vi "BinCoincidence.vi"(2 "lateral peaks":u32, 3 "rawdata":T1, 4 "center peak (µs)":dbl format="%.2f", 5 "delay channel":i32, 6 "histogram lenght (µs)":dbl format="%.2f", 7 "binning":dbl format="%.2f") -> (0 "center peak trace":u32[](array[numeric]), 1 "coincidence trace":dbl[](array[numeric]) format="%.2f")   [LabVIEW 2009]
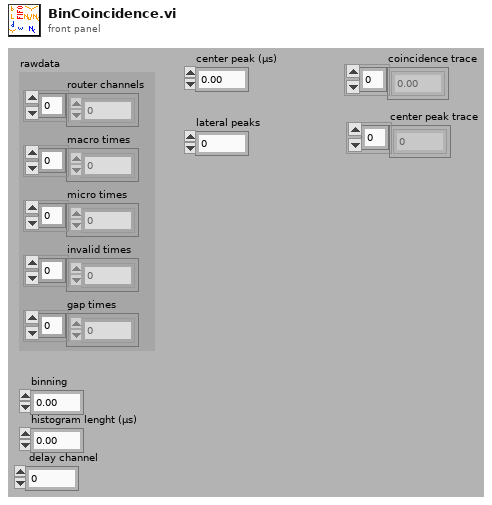
[diagram p1: front panel]
types:
  T1 = cluster{"router channels":u8[], "macro times":u32[], "micro times":u16[], "invalid times":u32[], "gap times":u32[]}
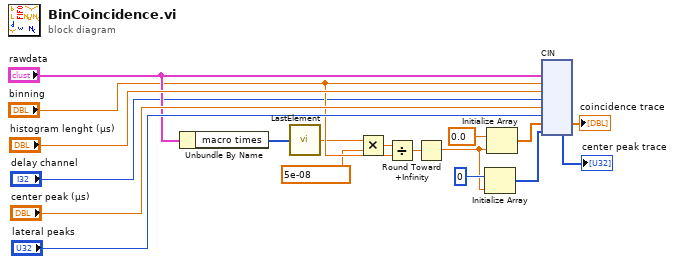
[diagram p0: block diagram]
diagram:
  n1 = Unbundle By Name("rawdata") -> ("macro times"=w12:u32[])
  n2 = call "LastElement.vi"("array"=w12) -> ("Numeric"=w7:dbl)
  n3 = Multiply(x=w7, y=5e-08) -> (x*y=w5:dbl)
  n4 = Divide(x=w5, y="binning") -> (x/y=w10:dbl)
  n5 = Round Toward +Infinity(x=w10) -> (ceil(x): smallest int >= x=w3:dbl)
  n6 = Initialize Array(u32 0 ("element"), w3) -> (w2:u32[])
  n7 = Initialize Array(0.0 ("element"), w3) -> (w9:dbl[])
  n8 = cin("rawdata", "binning", "histogram lenght (µs)", "delay channel", "center peak (µs)", "lateral peaks", w9, w2) -> (→"coincidence trace":dbl[], →"center peak trace":u32[])  [unwired: 6 in]
